vi "get_next_block_size.vi"(8 "error in (no error)":errorcluster, 11 "GenericDAQ in":refnum<class "GenericDAQ.lvclass">) -> (0 "error out":errorcluster, 2 "current block size":i32, 3 "GenericDAQ out":refnum<class "GenericDAQ.lvclass">)   [LabVIEW 2010, in "GenericDAQ.lvclass"]
uses:
  GenericDAQ.lvclass
  common/classes/GenericComponent/GenericComponent/class_data.vi
  common/classes/GenericComponent/GenericComponent/GenericComponent.lvclass
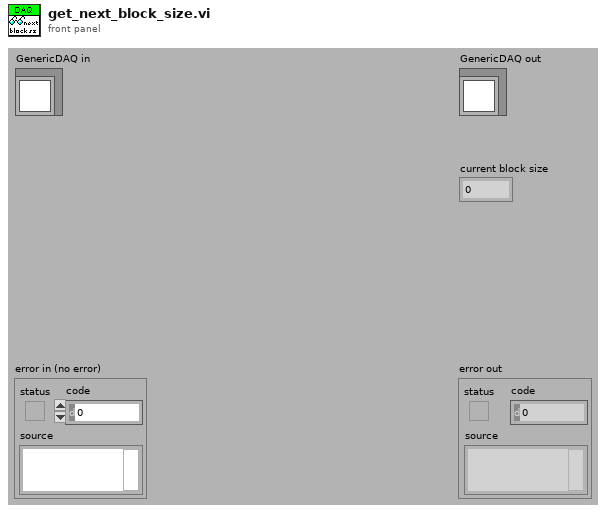
[diagram p1: front panel]
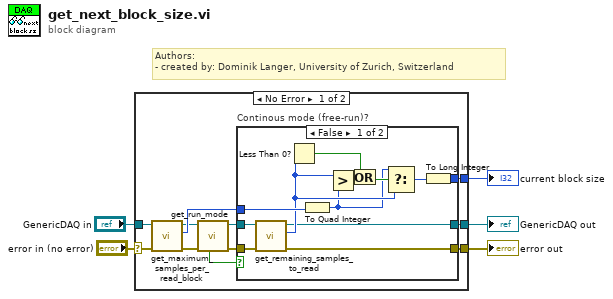
[diagram p0: block diagram]
diagram:
  # "Authors: \n- created by: Dominik Langer, University of Zurich, Switzerland"
  n1 = case shown="No Error" "error in (no error)" {
    selector: "error in (no error)" -> [w14 w33]
    tunnel: [w8 w33] -> w4
    tunnel: [w7 w32] -> w2
    tunnel: "GenericDAQ in" -> [w13 w32]
    tunnel: [w16 _] -> w1
    frame No Error {
      n2 = call-dynamic "get_maximum_samples_per_read_block.vi"("error in (no error)"=w14, "GenericDAQ.lvclass in"=w13) -> ("error out"=w12:errorcluster, "maximum samples per block"=w15:i32, "GenericDAQ.lvclass out"=w11:refnum<class "GenericDAQ.lvclass">)  [unwired: 7 out]
      n3 = call "get_run_mode.vi"("error in (no error)"=w12, "GenericPlugin in"=w11) -> ("error out"=w10:errorcluster, "GenericPlugin out"=w9:refnum<class "GenericDAQ.lvclass">, "is free run?"=w6:bool)  [unwired: 5 in, 2 out]
      n4 = case "Continous mode (free-run)?" shown="False" w6 {
        tunnel: [w27 w31] -> w16
        tunnel: w15 -> [w23 w31]
        tunnel: w10 -> [w20 w30]
        tunnel: w9 -> [w19 w29]
        tunnel: [w18 w30] -> w8
        tunnel: [w17 w29] -> w7
        frame False {
          n5 = call-dynamic "get_remaining_samples_to_read.vi"("error in (no error)"=w20, "GenericDAQ in"=w19) -> ("error out"=w18:errorcluster, "remaining samples to read"=w22:i64, "GenericDAQ out"=w17:refnum<class "GenericDAQ.lvclass">)  [unwired: 7 out]
          n6 = Less Than 0?(x=w22) -> (x < 0?=w25:bool)
          n7 = To Quad Integer(1:w23) -> (0:w21:i64)
          n8 = Greater?(x=w22, y=w21) -> (0:w26:bool)
          n9 = Or(x=w25, y=w26) -> (x .or. y?=w24:bool)
          n10 = Select(t=w21, s=w24, f=w22) -> (s? t:f=w28:i64)
          n11 = To Long Integer(number=w28) -> (32bit integer=w27:i32)
        }
        frame True {
        }
      }
    }
    frame Error {
    }
  }
  "error out" <- w4
  "GenericDAQ out" <- w2
  "current block size" <- w1
